vi "mod_movetoLatLon.vi"(0 "3D Eye":refnum<k7>, 1 "millisecond multiple":u32=20, 5 "Latitude Endpoint":dbl=45.0, 7 "Longitude Endpoint":dbl=45.0, 9 "Latitude Divisor":dbl=5.0, 11 "error in (no error)":errorcluster, 12 "Longitude Divisor":dbl=5.0) -> (4 "3D Eye out":refnum<k7>, 15 "error out":errorcluster)   [LabVIEW 2020, in "niDMT.lvlib"]
uses:
  <vilib>/addons/Modulation/niDMT.lvlib
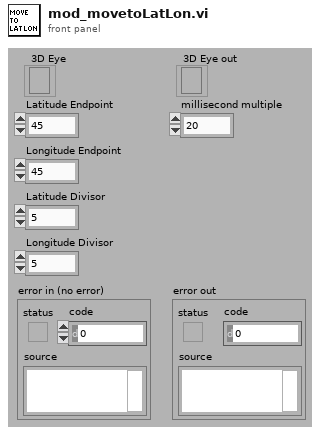
[diagram p1: front panel]
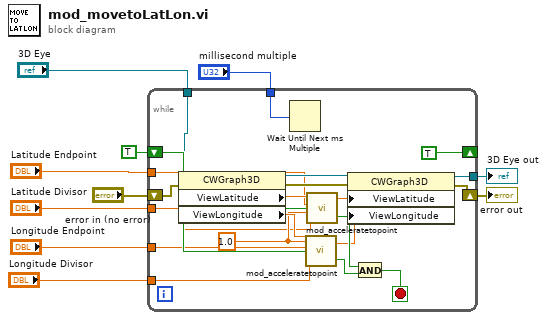
[diagram p0: block diagram]
diagram:
  n1 = while {
    shift-right: [TRUE] -> _
    shift-left: TRUE -> [w28]
    tunnel: "3D Eye" -> [w20]
    tunnel: "Latitude Endpoint" -> [w18]
    tunnel: "Longitude Endpoint" -> [w17]
    tunnel: "Longitude Divisor" -> [w16]
    tunnel: "Latitude Divisor" -> [w15]
    tunnel: "millisecond multiple" -> [w14]
    tunnel: [w13] -> w3
    shift-right: [w12] -> w2
    shift-left: "error in (no error)" -> [w11]
    stop <- w25 stop-if-true
    w19 = 1.0 ("tolerance")
    n2 = property class="CWGraph3D"(reference=w20, error in=w11) -> (reference out=w23:refnum<k7>, error out=w24:errorcluster, "ViewLatitude"=w30:dbl, "ViewLongitude"=w29:dbl)
    n3 = Wait Until Next ms Multiple(millisecond multiple=w14) -> ()  [unwired: 1 out]
    n4 = call <vilib>:"mod_acceleratetopoint.vi"("Startpoint"=w29, "Endpoint"=w17, "tolerance"=w19, "divisor"=w16, "reset? (F)"=w28) -> ("Next Point"=w21:dbl, "move complete"=w26:bool)
    n5 = call <vilib>:"mod_acceleratetopoint.vi"("Startpoint"=w30, "Endpoint"=w18, "tolerance"=w19, "divisor"=w15, "reset? (F)"=w28) -> ("Next Point"=w22:dbl, "move complete"=w27:bool)
    n6 = property class="CWGraph3D"(reference=w23, error in=w24, "ViewLatitude"=w22, "ViewLongitude"=w21) -> (reference out=w13:refnum<k7>, error out=w12:errorcluster)
    n7 = And(x=w27, y=w26) -> (x .and. y?=w25:bool)
  }
  "3D Eye out" <- w3
  "error out" <- w2
